vi "DSF.Memory.Buffer.Set Buffer Config.vi"(8 "error in (no error)":errorcluster, 10 "Buffer Config":refnum<class "DSF.Memory.Buffer.Config.lvclass">, 11 "Buffer in":refnum<class "DSF.Memory.Buffer.lvclass">) -> (0 "error out":errorcluster, 3 "Buffer out":refnum<class "DSF.Memory.Buffer.lvclass">)   [LabVIEW 2016, in "DSF.Memory.lvlib" / "DSF.Memory.Buffer.lvclass"]
uses:
  DSF.Memory.Buffer.lvclass
  DSF.Memory.Buffer.Config.lvclass
  DSF.Memory.Buffer.lvclass/DSF.Memory.Buffer.ctl
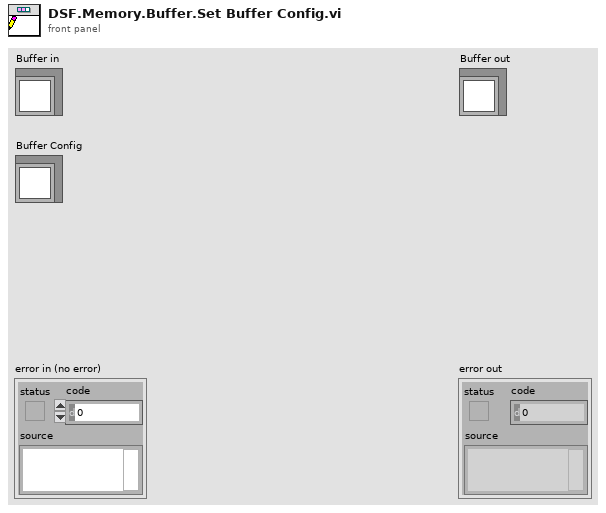
[diagram p1: front panel]
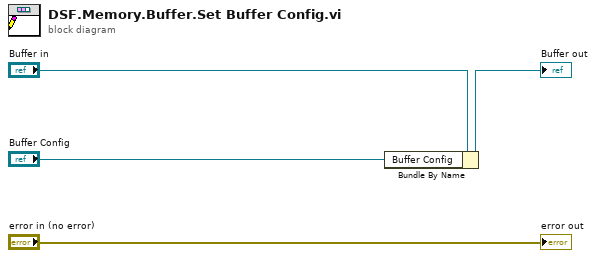
[diagram p0: block diagram]
diagram:
  n1 = Bundle By Name(cluster="Buffer in", "Buffer Config"="Buffer Config") -> (→"Buffer out":refnum<class "DSF.Memory.Buffer.lvclass">)
  "error out" <- "error in (no error)"
